vi "Open Workbook.vi"(8 "error in (no error)":errorcluster, 10 "File Path (last path)":path, 11 "Excel in":refnum<class "Excel.lvclass">) -> (0 "error out":errorcluster, 3 "Excel out":refnum<class "Excel.lvclass">)   [LabVIEW 2016, in "Excel.lvclass"]
uses:
  Excel.lvclass
  Excel.lvclass/Excel.ctl
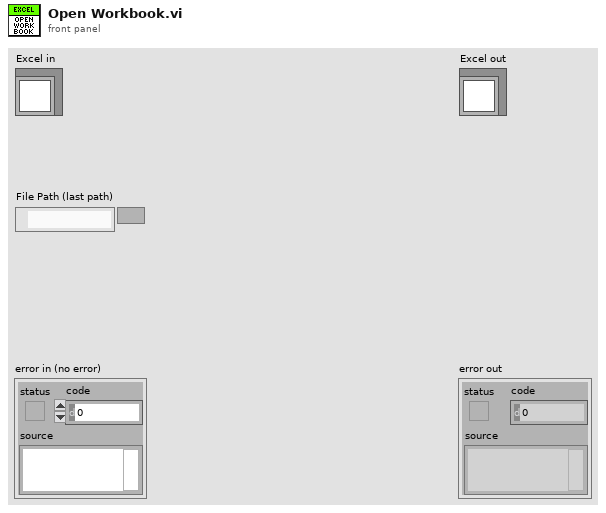
[diagram p1: front panel]
types:
  T1 = enum16{"Open Existing", "Open Active", "Open New", "Cancelled"}
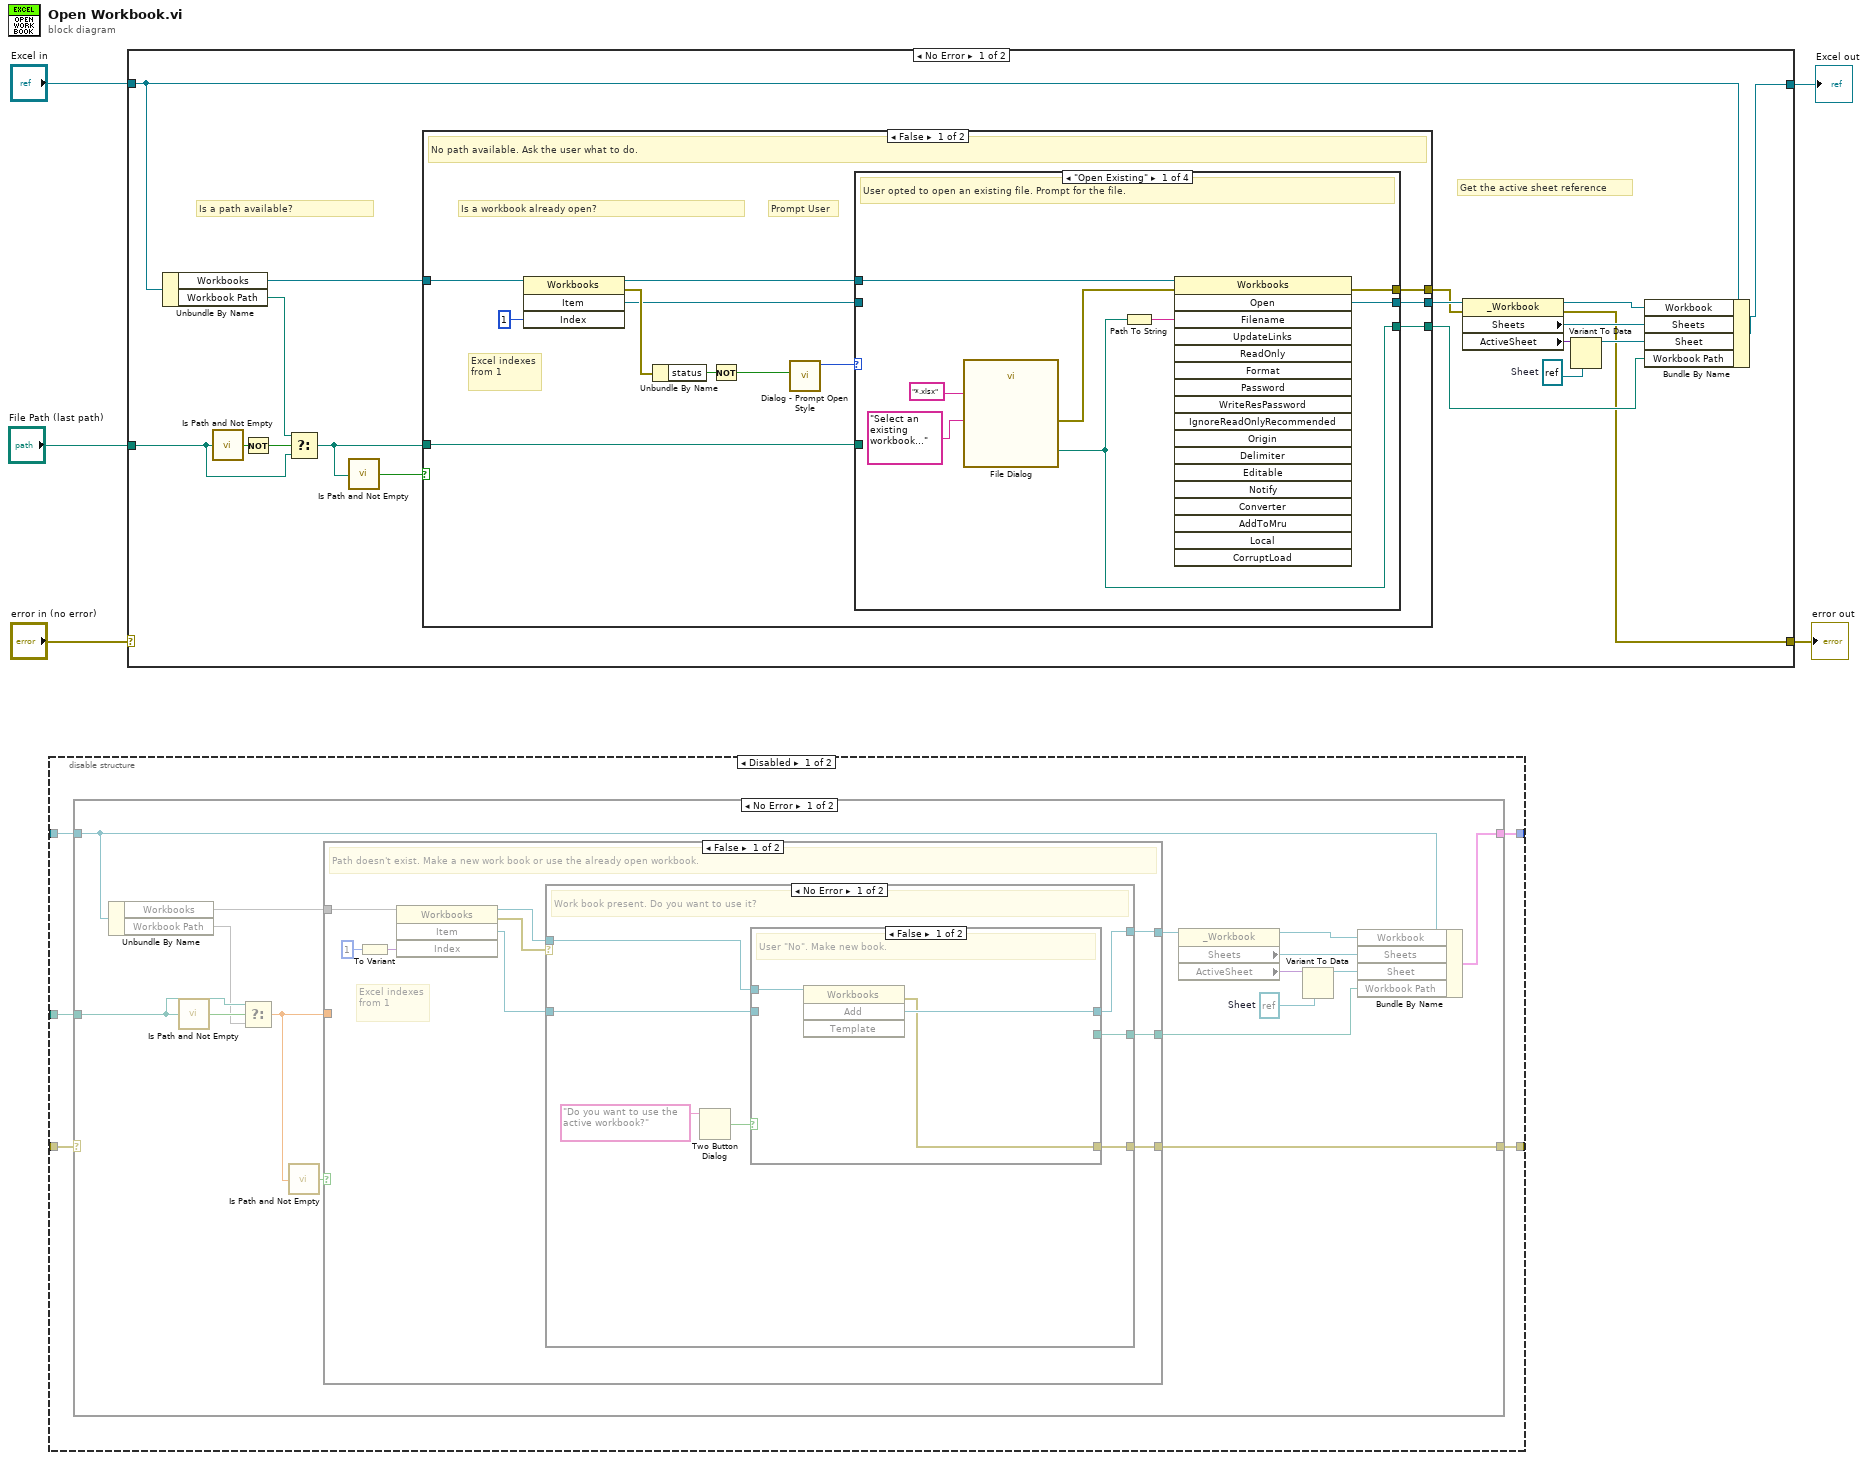
[diagram p0: block diagram]
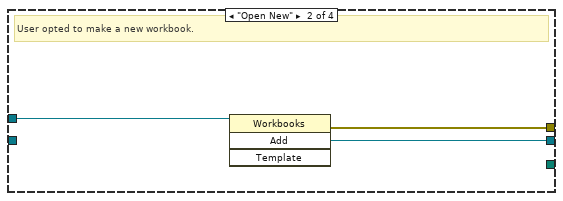
[diagram p2: hidden frame]
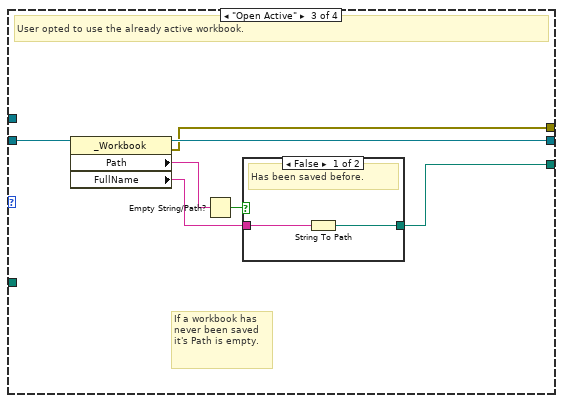
[diagram p3: hidden frame]
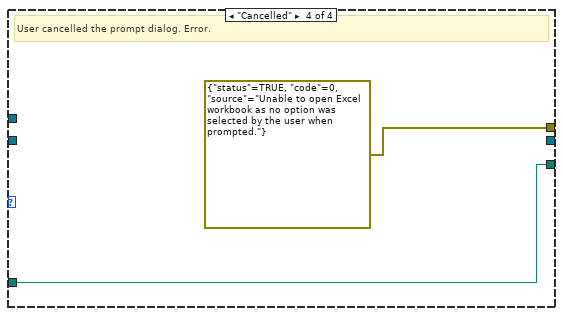
[diagram p5: hidden frame]
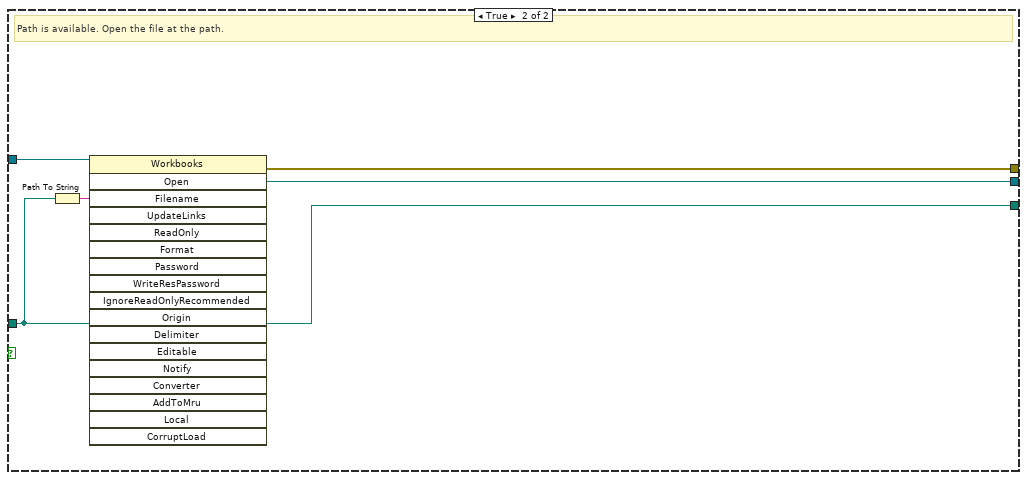
[diagram p6: hidden frame]
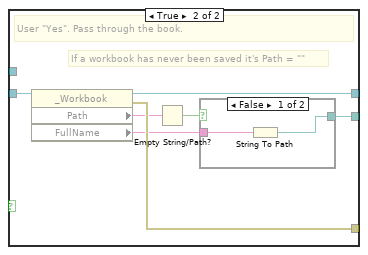
[diagram p8: hidden frame]
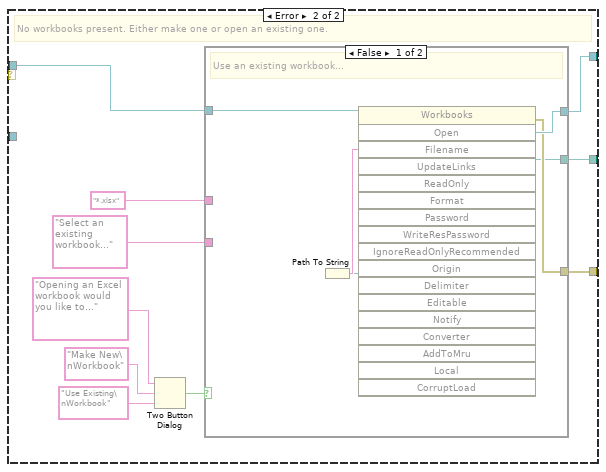
[diagram p10: hidden frame]
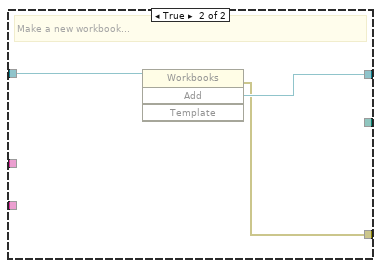
[diagram p11: hidden frame]
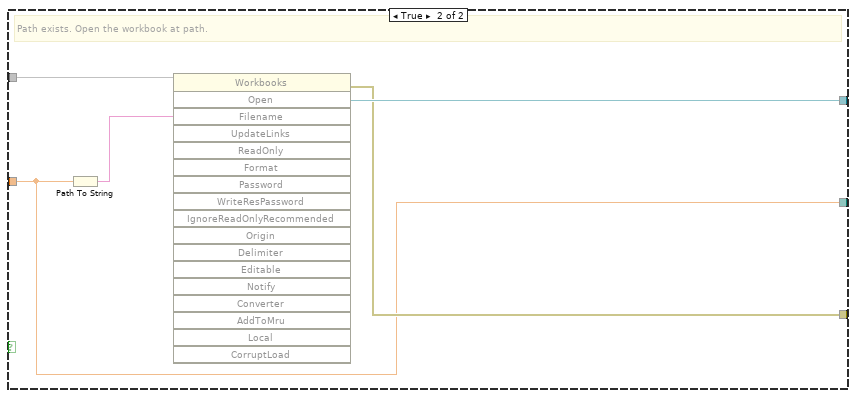
[diagram p12: hidden frame]
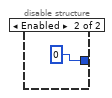
[diagram p14: hidden frame]
diagram:
  n1 = disable-structure shown="Disabled" {
    disable-tunnel: _ -> [w10 _]
    disable-tunnel: [w9 _] -> _
    disable-tunnel: _ -> [w8 _]
    disable-tunnel: [w7 0] -> _
    disable-tunnel: _ -> [w6 _]
    frame Disabled {
      n2 = case shown="No Error" w10 {
        selector: w10 -> [_ w79]
        tunnel: [w23 w79] -> w9
        tunnel: [w24 w78] -> w7
        tunnel: w8 -> [w25 w78]
        tunnel: w6 -> [w15 _]
        frame No Error {
          w17 = refnum<k7> refnum  # Sheet
          n3 = Unbundle By Name(w25) -> ("Workbooks"=w26, "Workbook Path"=w14)
          n4 = call <vilib>:"Is Path and Not Empty.vi"("path"=w15) -> ("Is Path and Not Empty?"=w16:bool)  [unwired: 4 in]
          n5 = Select(t=w15, s=w16, f=w14) -> (s? t:f=w13:dbl)
          n6 = call <vilib>:"Is Path and Not Empty.vi"("path"=w13) -> ("Is Path and Not Empty?"=w12:bool)  [unwired: 4 in]
          n7 = case shown="False" w12 {
            tunnel: w26 -> [w34 w77]
            tunnel: [w35 w76] -> w22
            tunnel: w13 -> [_ w73]
            tunnel: [w31 w75] -> w23
            tunnel: [w27 w73] -> w11
            frame False {
              # "Excel indexes from 1"
              # "Path doesn't exist. Make a new work book or use the already open workbook."
              n8 = To Variant(anything=1) -> (Variant=w33:variant)
              n9 = invoke class="Workbooks" method="Item"(reference=w34, "Index"=w33) -> (reference out=w30:refnum<k7>, error out=w28:errorcluster, "Item"=w29:refnum<k7>)  [unwired: 2 in, 1 out]
              n10 = case shown="No Error" w28 {
                tunnel: [w39 w59] -> w35
                tunnel: [w37 w58] -> w31
                tunnel: w30 -> [w38 w60]
                tunnel: w29 -> [w40 _]
                tunnel: [w36 w55] -> w27
                frame No Error {
                  # "Work book present. Do you want to use it?"
                  n11 = Two Button Dialog(message="Do you want to use the active workbook?") -> (T button?=w41:bool)  [unwired: 2 in]
                  n12 = case shown="False" w41 {
                    tunnel: w40 -> [_ w52]
                    tunnel: [w44 w51] -> w39
                    tunnel: w38 -> [w45 _]
                    tunnel: [w43 w50] -> w37
                    tunnel: [_ w46] -> w36
                    frame False {
                      # "User \"No\". Make new book."
                      n13 = invoke class="Workbooks" method="Add"(reference=w45) -> (error out=w43:errorcluster, "Add"=w44:refnum<k7>)  [unwired: 3 in, 2 out]
                    }
                    frame True {
                      # "If a workbook has never been saved it's Path = \"\""
                      # "User \"Yes\". Pass through the book."
                      n14 = property class="_Workbook"(reference=w52) -> (reference out=w51:refnum<k7>, error out=w50:errorcluster, "Path"=w49:string, "FullName"=w47:string)  [unwired: 1 in]
                      n15 = Empty String/Path?(string/path=w49) -> (empty?=w48:bool)
                      n16 = case shown="False" w48 {
                        tunnel: w47 -> [w54 _]
                        tunnel: [w53 _] -> w46
                        frame False {
                          n17 = String To Path(string=w54) -> (path=w53:path)
                        }
                        frame True {
                        }
                      }
                    }
                  }
                }
                frame Error {
                  # "No workbooks present. Either make one or open an existing one."
                  n18 = Two Button Dialog(message="Opening an Excel workbook would you like to...", 1:"Use Existing\nWorkbook" ("F button name (\"Cancel\")"), 2:"Make New\nWorkbook" ("T button name (\"OK\")")) -> (T button?=w61:bool)
                  n19 = case shown="False" w61 {
                    tunnel: w60 -> [w68 w72]
                    tunnel: [w69 w71] -> w59
                    tunnel: [w66 w70] -> w58
                    tunnel: "Select an existing workbook..." ("pattern (all files)") -> [_ _]
                    tunnel: "*.xlsx" ("pattern (all files)") -> [_ _]
                    tunnel: [w65 _] -> w55
                    frame False {
                      # "Use an existing workbook..."
                      n20 = Path To String() -> (path=w65:path, string=w67:string)
                      n21 = invoke class="Workbooks" method="Open"(reference=w68, "Filename"=w67) -> (error out=w66:errorcluster, "Open"=w69:refnum<k7>)  [unwired: 16 in, 16 out]
                    }
                    frame True {
                      # "Make a new workbook..."
                      n22 = invoke class="Workbooks" method="Add"(reference=w72) -> (error out=w70:errorcluster, "Add"=w71:refnum<k7>)  [unwired: 3 in, 2 out]
                    }
                  }
                }
              }
            }
            frame True {
              # "Path exists. Open the workbook at path."
              n23 = Path To String(path=w73) -> (string=w74:string)
              n24 = invoke class="Workbooks" method="Open"(reference=w77, "Filename"=w74) -> (error out=w75:errorcluster, "Open"=w76:refnum<k7>)  [unwired: 16 in, 16 out]
            }
          }
          n25 = property class="_Workbook"(reference=w22) -> (reference out=w21:refnum<k7>, "Sheets"=w20:refnum<k7>, "ActiveSheet"=w19:variant)  [unwired: 1 in, 1 out]
          n26 = Variant To Data(type=w17, Variant=w19) -> (data=w18:refnum<k7>)  [unwired: 1 in, 1 out]
          n27 = Bundle By Name(cluster=w25, "Workbook"=w21, "Sheets"=w20, "Sheet"=w18, "Workbook Path"=w11) -> (w24:cluster{})
        }
        frame Error {
        }
      }
    }
    frame Enabled {
    }
  }
  n28 = case shown="No Error" "error in (no error)" {
    selector: "error in (no error)" -> [_ w139]
    tunnel: "Excel in" -> [w83 w138]
    tunnel: "File Path (last path)" -> [w95 _]
    tunnel: [w82 w138] -> w2
    tunnel: [w81 w139] -> w1
    frame No Error {
      w91 = refnum<k7> refnum  # Sheet
      # "Get the active sheet reference"
      # "Is a path available?"
      n29 = Unbundle By Name(w83) -> ("Workbooks"=w94:refnum<k7>, "Workbook Path"=w96:path)
      n30 = call <vilib>:"Is Path and Not Empty.vi"("path"=w95) -> ("Is Path and Not Empty?"=w98:bool)  [unwired: 4 in]
      n31 = Not(x=w98) -> (.not. x?=w97:bool)
      n32 = Select(t=w96, s=w97, f=w95) -> (s? t:f=w92:path)
      n33 = call <vilib>:"Is Path and Not Empty.vi"("path"=w92) -> ("Is Path and Not Empty?"=w93:bool)  [unwired: 4 in]
      n34 = case shown="False" w93 {
        tunnel: w94 -> [w110 w137]
        tunnel: w92 -> [w99 w134]
        tunnel: [w102 w135] -> w86
        tunnel: [w101 w134] -> w84
        tunnel: [w100 w133] -> w85
        frame False {
          # "Prompt User"
          # "Is a workbook already open?"
          # "Excel indexes from 1"
          # "No path available. Ask the user what to do."
          n35 = invoke class="Workbooks" method="Item"(reference=w110, "Index"=1) -> (reference out=w104:refnum<k7>, error out=w108:errorcluster, "Item"=w103:refnum<k7>)  [unwired: 2 in, 1 out]
          n36 = Unbundle By Name(w108) -> ("status"=w107:bool)
          n37 = Not(x=w107) -> (.not. x?=w106:bool)
          n38 = call "Dialog - Prompt Open Style.vi"("Include active book option?"=w106) -> ("Open Style"=w105:T1)  [unwired: 9 in, 1 out]
          n39 = case shown="\"Open Existing\"" w105 {
            tunnel: w104 -> [w118 w121 _ _]
            tunnel: w103 -> [_ _ w128 _]
            tunnel: [w113 w119 w127 _] -> w102
            tunnel: [w112 _ w123 w132] -> w101
            tunnel: [w111 w120 w122 errorcluster {"status"=TRUE, "code"=0, "source"="Unable to open Excel workbook as no option was selected by the user when prompted."} ("error constant")] -> w100
            tunnel: w99 -> [_ _ _ w132]
            frame "Open Existing" {
              # "User opted to open an existing file. Prompt for the file."
              n40 = call "File Dialog"("prompt"="Select an existing workbook..." ("pattern (all files)"), "pattern (all files)"="*.xlsx") -> ("selected path"=w112:path, "error out"=w114:errorcluster)  [unwired: 10 in, 2 out]
              n41 = Path To String(path=w112) -> (string=w115:string)
              n42 = invoke class="Workbooks" method="Open"(reference=w118, error in=w114, "Filename"=w115) -> (error out=w111:errorcluster, "Open"=w113:refnum<k7>)  [unwired: 15 in, 16 out]
            }
            frame "Open New" {
              # "User opted to make a new workbook."
              n43 = invoke class="Workbooks" method="Add"(reference=w121) -> (error out=w120:errorcluster, "Add"=w119:refnum<k7>)  [unwired: 3 in, 2 out]
            }
            frame "Open Active" {
              # "If a workbook has never been saved it's Path is empty."
              # "User opted to use the already active workbook."
              n44 = property class="_Workbook"(reference=w128) -> (reference out=w127:refnum<k7>, error out=w122:errorcluster, "Path"=w126:string, "FullName"=w124:string)  [unwired: 1 in]
              n45 = Empty String/Path?(string/path=w126) -> (empty?=w125:bool)
              n46 = case shown="False" w125 {
                tunnel: w124 -> [w130 _]
                tunnel: [w129 _] -> w123
                frame False {
                  # "Has been saved before."
                  n47 = String To Path(string=w130) -> (path=w129:path)
                }
                frame True {
                  # "Has never been saved."
                }
              }
            }
            frame "Cancelled" {
              # "User cancelled the prompt dialog. Error."
            }
          }
        }
        frame True {
          # "Path is available. Open the file at the path."
          n48 = Path To String(path=w134) -> (string=w136:string)
          n49 = invoke class="Workbooks" method="Open"(reference=w137, "Filename"=w136) -> (error out=w133:errorcluster, "Open"=w135:refnum<k7>)  [unwired: 16 in, 16 out]
        }
      }
      n50 = property class="_Workbook"(reference=w86, error in=w85) -> (reference out=w87:refnum<k7>, error out=w81:errorcluster, "Sheets"=w88:refnum<k7>, "ActiveSheet"=w89:variant)
      n51 = Variant To Data(type=w91, Variant=w89) -> (data=w90:refnum<k7>)  [unwired: 1 in, 1 out]
      n52 = Bundle By Name(cluster=w83, "Workbook"=w87, "Sheets"=w88, "Sheet"=w90, "Workbook Path"=w84) -> (w82:refnum<class "Excel.lvclass">)
    }
    frame Error {
    }
  }
  "error out" <- w1
  "Excel out" <- w2
